vi "Process Ch1.vi"() -> (2 "Max1":u32, 3 "Max0":u32)   [LabVIEW 2016]
uses:
  <vilib>/rvi/Emulation/niFpgaGetClockAttributes.vi
  <vilib>/rvi/Emulation/niFpgaSctlEmulationGetInTimedLoop.vi
  <vilib>/rvi/Emulation/niFpgaEmulationReportErrorSimple.vi
  <vilib>/rvi/Emulation/niFpgaEmulationIsFPGAContextNoSignature.vi
  <vilib>/rvi/DataTransferAndStorage/Container/Common/niFpgaContainerGetUniqueNameForEmu.vi
  <vilib>/rvi/Memory/Memory_Emulation/niFpgaMemoryEmulationCacheClearOnFirstRun.vi
  <vilib>/rvi/Memory/Memory_Emulation/nirvimemoryEmulationManagerCache_MakeExclusive.vi
  <vilib>/rvi/Memory/Memory_Emulation/niFpgaMemoryEmulationValidateCache.vi
  <vilib>/rvi/Memory/Memory_Emulation/nirvimemoryEmulationManagerCache_InsertValue.vi
  <vilib>/Utility/error.llb/Clear Errors.vi
  <vilib>/rvi/Memory/Memory_Emulation/nirvimemoryEmulationManagerCache_ReleaseExclusive.vi
  <vilib>/rvi/Memory/Memory_Emulation/nirvimemoryEmulationManagerCache_GetValue.vi
  <vilib>/rvi/Memory/Memory_Emulation/nirvimemoryEmulationManagerCache_SetValue.vi
  <vilib>/rvi/Emulation/niFpgaProcessEmulError.vi
  <vilib>/rvi/FIFO/Fifo_Resource/nirvififoEmulationSetSize.vi
  <vilib>/rvi/FIFO/Fifo_Resource/nirviFifoEmulationQueueMgr.vi
  <instcachedir>/0/nirviFifoEmulationQueueMgr_E5CAEC123FF24DC58D834DCA3CDAA9B5.lvgen/nirviFifoEmulationQueueMgr_E5CAEC123FF24DC58D834DCA3CDAA9B5_001.vi
  <vilib>/rvi/errors/niFpgaSetErrorForExecOnDevCompSimple.vi
  <vilib>/rvi/eio/common/nirviEmuReportErrorAndStop.vi
  <vilib>/rvi/FIFO/Fifo_Resource/nirvififoEmulationCreateLock.vi
  <vilib>/rvi/FIFO/Fifo_Resource/nirvififoEmulationObtainLock.vi
  <vilib>/rvi/FIFO/Fifo_Resource/nirvififoEmulationReleaseLock.vi
  <vilib>/rvi/occurrence/nirviWaitOnOccurrenceBase.vi
  <vilib>/rvi/errors/nirviReportUnexpectedCaseInternalError.vi
  <vilib>/rvi/errors/nirviReportUnexpectedCaseInternalError (U32).vi
  <vilib>/rvi/Memory/Memory_Emulation/nirvimemoryFastEmulation.vi
  <vilib>/rvi/Memory/Memory_Emulation/nirvimemoryEmulation.vi
  <vilib>/rvi/Emulation/niFpgaCriticalErrorInLSC.vi
  <vilib>/rvi/DataTransferAndStorage/Container/XNode/niFpgaContainer.xnode
  <vilib>/rvi/DataTransferAndStorage/Register/Emulation/niFpgaRegisterEmulation.vi
  <vilib>/rvi/FIFO/Fifo_Resource/nirvififoEmulationGetNumberOfElementsToRead.vi
  <vilib>/rvi/FIFO/Fifo_Resource/nirvififoEmulationRead.vi
  <vilib>/rvi/FXPMathLib/FxpAdd/XNode/nifxpmath_Add.xnode
  <vilib>/rvi/FXPMathLib/FxpSub/XNode/nifxpmath_Sub.xnode
  <vilib>/rvi/FXPMathLib/sim/FxpSim.dll
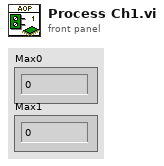
[diagram p1: front panel]
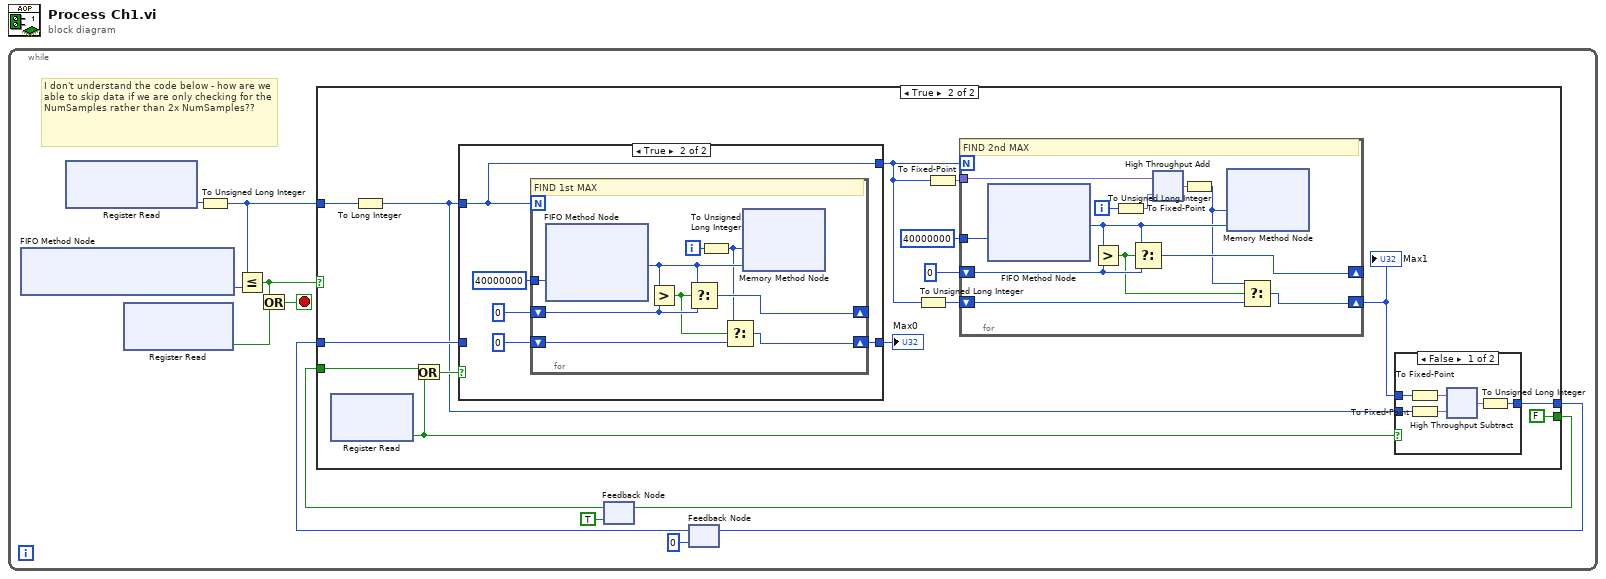
[diagram p0: block diagram]
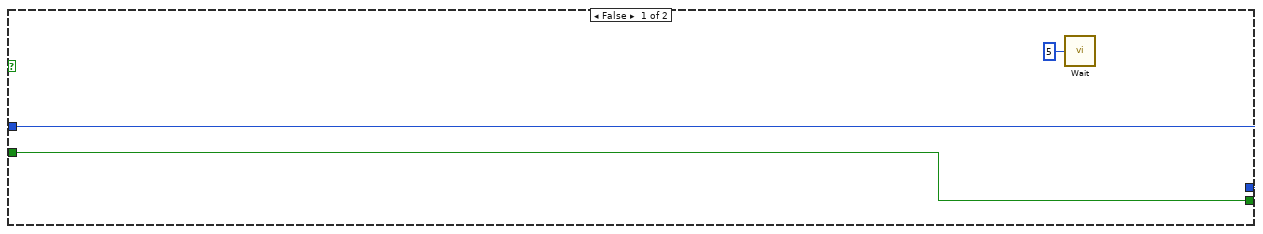
[diagram p2: hidden frame]
diagram:
  n1 = while {
    stop <- w4 stop-if-true
    # "I don't understand the code below - how are we able to skip data if we are only checking for the NumSamples rather than 2x NumSamples??"
    n2 = xnode ("FIFO Method Node")() -> ("Number of Elements to Read"=w12:u32)  [unwired: 1 in, 1 out]
    n3 = xnode ("Register Read")() -> ("Data"=w2:u16)  [unwired: 1 in, 1 out]
    n4 = xnode ("Register Read")() -> ("Data"=w5:bool)  [unwired: 1 in, 1 out]
    n5 = To Unsigned Long Integer(number=w2) -> (unsigned 32bit integer=w1:u32)
    n6 = Less Or Equal?(x=w1, y=w12) -> (x <= y?=w6:bool)
    n7 = Or(x=w6, y=w5) -> (x .or. y?=w4:bool)
    n8 = feedback #1(TRUE) -> (w9:bool)
    n9 = feedback #2(u32 0) -> (w8:u32)
    n10 = case shown="True" w6 {
      tunnel: w1 -> [_ w30]
      tunnel: w8 -> [w15 w29]
      tunnel: [w15 w28] -> w3
      tunnel: w9 -> [w14 w24]
      tunnel: [w14 FALSE] -> w11
      frame False {
        n11 = call "Wait"("Count(uSec)"=u32 5) -> ()  [unwired: 1 out]
      }
      frame True {
        n12 = xnode ("Register Read")() -> ("Data"=w22:bool)  [unwired: 1 in, 1 out]
        n13 = To Long Integer(number=w30) -> (32bit integer=w18:i32)
        n14 = Or(x=w24, y=w22) -> (x .or. y?=w23:bool)
        n15 = case shown="True" w23 {
          tunnel: [w38 w43] -> w16
          tunnel: w18 -> [w37 w39]
          tunnel: w29 -> [w38 _]
          tunnel: [w37 w39] -> w17
          frame False {
          }
          frame True {
            n16 = for {
              N: w39 -> [_]
              shift-right: [w50] -> _
              shift-left: i16 0 ("Element") -> [w51]
              shift-right: [w47] -> w43
              shift-left: u32 0 ("Element") -> [w48]
              tunnel: 40000000 ("Timeout") -> [w44]
              i -> [w46]
              # "FIND 1st MAX"
              n17 = xnode ("FIFO Method Node")("Timeout"=w44) -> ("Element"=w52:i16)  [unwired: 1 in, 2 out]
              n18 = Greater?(x=w52, y=w51) -> (0:w49:bool)
              n19 = Select(t=w52, s=w49, f=w51) -> (s? t:f=w50:i16)
              n20 = To Unsigned Long Integer(number=w46) -> (unsigned 32bit integer=w45:u32)
              n21 = Select(t=w45, s=w49, f=w48) -> (s? t:f=w47:u32)
              n22 = xnode ("Memory Method Node")("Address"=w45, "Data"=w52) -> ()  [unwired: 1 in, 1 out]
            }
          }
        }
        "Max0" <- w16
        n23 = To Unsigned Long Integer(number=w17) -> (unsigned 32bit integer=w26:u32)
        n24 = To Fixed-Point(number=w17) -> (fixed-point=w25:fxp<+/-,32,32>)  [unwired: 1 in]
        n25 = for {
          N: w17 -> [_]
          shift-right: [w62] -> _
          shift-left: i16 0 ("Element") -> [w63]
          shift-right: [w59] -> w20
          shift-left: w26 -> [w60]
          tunnel: w25 -> [w56]
          tunnel: 40000000 ("Timeout") -> [w53]
          i -> [w57]
          # "FIND 2nd MAX"
          n26 = xnode ("FIFO Method Node")("Timeout"=w53) -> ("Element"=w64:i16)  [unwired: 1 in, 2 out]
          n27 = Greater?(x=w64, y=w63) -> (0:w61:bool)
          n28 = To Fixed-Point(number=w57) -> (fixed-point=w55:fxp<+/-,32,32>)  [unwired: 1 in]
          n29 = Select(t=w64, s=w61, f=w63) -> (s? t:f=w62:i16)
          n30 = xnode ("High Throughput Add")("x"=w56, "y"=w55) -> ("x+y"=w54:fxp<+,32,32>)
          n31 = To Unsigned Long Integer(number=w54) -> (unsigned 32bit integer=w58:u32)
          n32 = xnode ("Memory Method Node")("Address"=w58, "Data"=w64) -> ()  [unwired: 1 in, 1 out]
          n33 = Select(t=w58, s=w61, f=w60) -> (s? t:f=w59:u32)
        }
        "Max1" <- w20
        n34 = case shown="False" w22 {
          tunnel: [w34 _] -> w28
          tunnel: w20 -> [w32 _]
          tunnel: w18 -> [w31 _]
          frame False {
            n35 = To Fixed-Point(number=w32) -> (fixed-point=w36:fxp<+,32,32>)  [unwired: 1 in]
            n36 = To Fixed-Point(number=w31) -> (fixed-point=w33:fxp<+/-,32,32>)  [unwired: 1 in]
            n37 = xnode "High Throughput Subtract"("x"=w36, "y"=w33) -> ("x-y"=w35:fxp<+,32,32>)
            n38 = To Unsigned Long Integer(number=w35) -> (unsigned 32bit integer=w34:u32)
          }
          frame True {
          }
        }
      }
    }
    n39 = feedback-in #1(w11) -> ()
    n40 = feedback-in #2(w3) -> ()
  }
